vi "ImageClickDetect V0.1.vi"(5 "Change":refnum<vi>, 7 "Stop":refnum<vi>, 9 "Mouse Point":refnum<vi>, 11 "image Ref String":string) -> ()   [LabVIEW 2014]
panel:
  out "ImXY_Point":i32[](array[numeric])
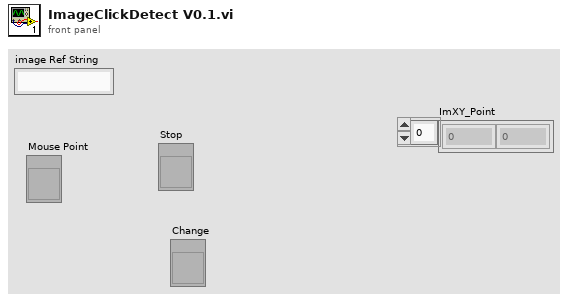
[diagram p1: front panel]
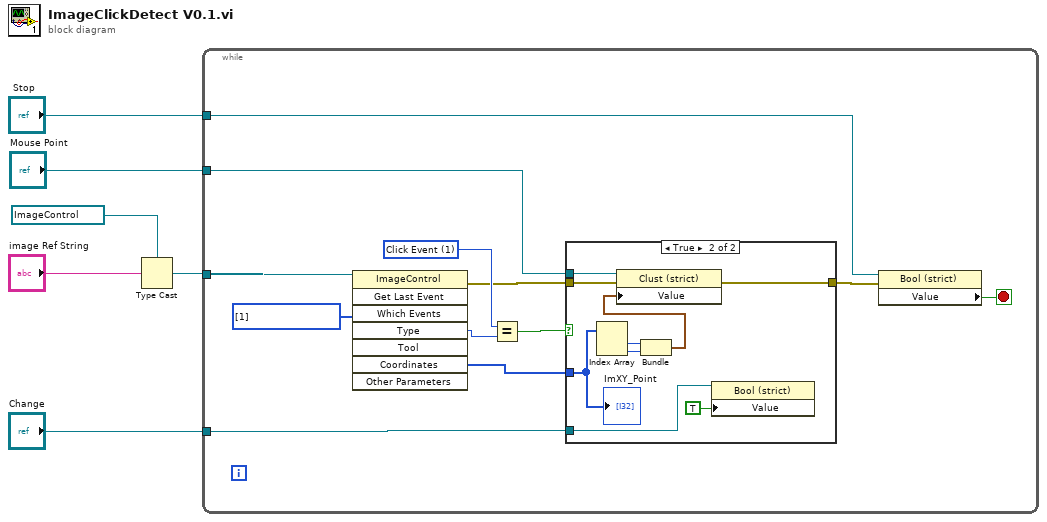
[diagram p0: block diagram]
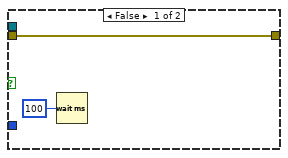
[diagram p2: hidden frame]
diagram:
  n1 = Type Cast(type=refnum<vi> refnum ("Image"), x="image Ref String") -> (*(type *) &x=w4:refnum<vi>)
  n2 = while {
    tunnel: w4 -> [w18]
    tunnel: "Stop" -> [w12]
    tunnel: "Mouse Point" -> [w10]
    tunnel: "Change" -> [w7]
    stop <- w11 stop-if-true
    w15 = 1 items=["No Event"=0, "Click Event"=1, "Draw Event"=2, "Size Event"=4, "Scroll Event"=5, "Double Click Event"=8]
    w17 = i32[] [1] items=["No Event"=0, "Click Event"=1, "Draw Event"=2, "Size Event"=4, "Scroll Event"=5, "Double Click Event"=8] ("Which Events")
    n3 = invoke class="ImageControl" method="Get Last Event"(reference=w18, "Which Events"=w17) -> (error out=w9:errorcluster, "Type"=w16:i32, "Coordinates"=w13:i32[])  [unwired: 6 in, 5 out]
    n4 = Equal?(x=w15, y=w16) -> (x = y?=w14:bool)
    n5 = case shown="True" w14 {
      tunnel: w13 -> [_ w25]
      tunnel: w10 -> [_ w29]
      tunnel: w9 -> [w19 w28]
      tunnel: [w19 w27] -> w8
      tunnel: w7 -> [_ w21]
      frame False {
        n6 = Wait (ms)(milliseconds to wait=u32 100) -> ()  [unwired: 1 out]
      }
      frame True {
        n7 = Index Array(array=w25) -> (element #1=w24:i32, element #2=w23:i32)  [unwired: 2 in]
        n8 = Bundle(w24, w23) -> (w26:cluster{i32, i32})  [unwired: 1 in]
        n9 = property class="Clust (strict)"(reference=w29, error in=w28, "Value"=w26) -> (error out=w27:errorcluster)  [unwired: 1 out]
        n10 = property class="Bool (strict)"(reference=w21, "Value"=TRUE ("Boolean")) -> ()  [unwired: 1 in, 2 out]
        "ImXY_Point" <- w25
      }
    }
    n11 = property class="Bool (strict)"(reference=w12, error in=w8) -> ("Value"=w11:bool)  [unwired: 2 out]
  }
